vi "test_RemoteFgenSession_CallCloseMeasurementLinkSessionWithDetachBehavior_RemoteSessionDetached.vi"(8 "error in":errorcluster) -> (0 "error out":errorcluster, 2 "result":string, 3 "pass":bool)   [LabVIEW 2020, in "MeasurementServerTests.lvlib"]
uses:
  MeasurementServerTests.lvlib
  Runtime/Sessions/niFGEN Sessions/Session Factory/Session Factory.lvclass
  Runtime/Sessions/Instrument Sessions/ISession Factory/Initialize and Close Session Behavior.ctl
  Runtime/Sessions/Instrument Sessions/ISession Factory/ISession Factory.lvclass
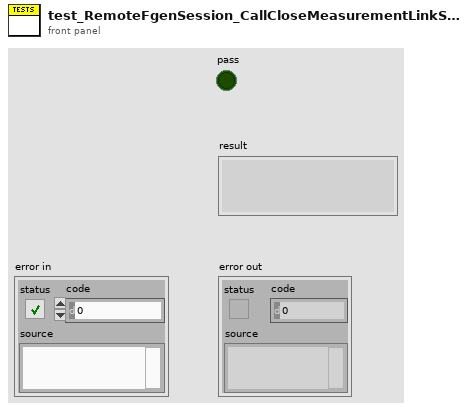
[diagram p1: front panel]
types:
  T1 = typedef "Plug-In SDK Instrument Sessions.lvlib/ISession Factory.lvclass/Remote Connection Options.ctl" = cluster{"session name":string, "address":string, "port":u32}
  T2 = typedef "Plug-In SDK Instrument Sessions.lvlib/ISession Factory.lvclass/Initialize and Close Session Behavior.ctl" = enum16{"Initialize and Close", "Attach and Detach", "Initialize and Detach", "Attach and Close"}
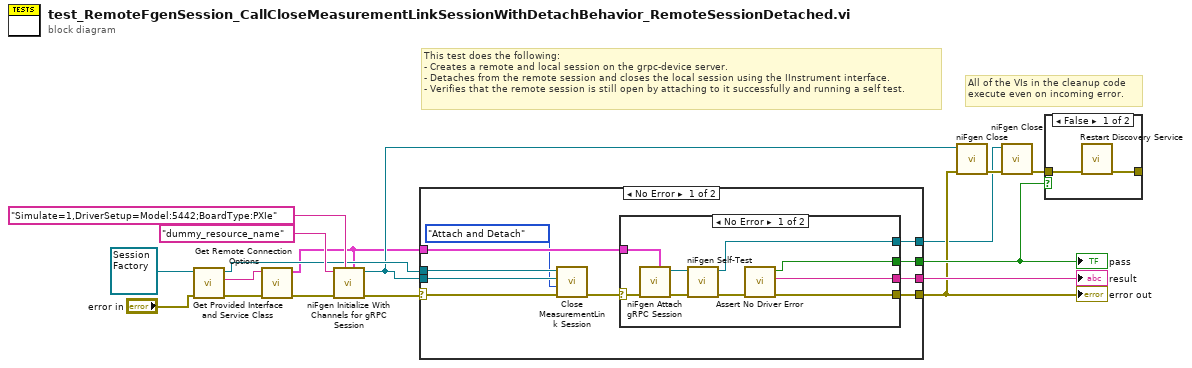
[diagram p0: block diagram]
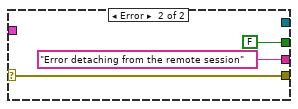
[diagram p2: hidden frame]
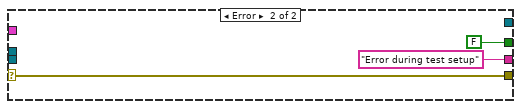
[diagram p3: hidden frame]
diagram:
  # "All of the VIs in the cleanup code\nexecute even on incoming error."
  # "This test does the following:\n- Creates a remote and local session on the grpc-device server.\n- Detaches from the remote session and closes the local session using the IInstrument interface.\n- Verifies that the remote session is still open by attaching to it successfully and running a self test."
  n1 = call-dynamic "Get Provided Interface and Service Class.vi"("error in"="error in", "session factory in"=refnum<class "Session Factory.lvclass"> refnum ("MeasurementLink niFGEN.lvlib:Instrument.lvclass")) -> ("error out"=w15:errorcluster, "provided interface"=w14:string, "session factory out"=w10:refnum<class "Session Factory.lvclass">)  [unwired: 6 in, 1 out]
  n2 = call "Get Remote Connection Options.vi"("error in"=w15, "provided interface"=w14) -> ("error out"=w16:errorcluster, "remote connection options"=w2:T1)  [unwired: 8 in]
  n3 = call <instrlib>:"niFgen Initialize With Channels for gRPC Session.vi"("gRPC Options"=w2, "Option String"="Simulate=1,DriverSetup=Model:5442;BoardType:PXIe" ("option string"), "error in (no error)"=w16, "Resource Name"="dummy_resource_name" ("resource name")) -> ("error out"=w11:errorcluster, "Instrument Handle Out"=w5:refnum<k15>)  [unwired: 6 in]
  n4 = case shown="No Error" w11 {
    selector: w11 -> [w27 w41]
    tunnel: w10 -> [w26 _]
    tunnel: w5 -> [w25 _]
    tunnel: w2 -> [w24 _]
    tunnel: [w22 w41] -> w4
    tunnel: [w21 FALSE] -> w6
    tunnel: [w20 "Error during test setup" ("f")] -> w9
    tunnel: [w18 _] -> w1
    frame No Error {
      n5 = call-dynamic "Close MeasurementLink Session.vi"("error in"=w27, "initialize and close session behavior"=Initialize_and_Close_Session_Behavior."Attach and Detach", "session in"=w25, "session factory in"=w26) -> ("error out"=w23:errorcluster)  [unwired: 7 in]
      n6 = case shown="No Error" w23 {
        selector: w23 -> [w36 w37]
        tunnel: w24 -> [w33 _]
        tunnel: [w28 w37] -> w22
        tunnel: [w30 FALSE] -> w21
        tunnel: [w29 "Error detaching from the remote session" ("f")] -> w20
        tunnel: [w32 _] -> w18
        frame No Error {
          n7 = call <instrlib>:"niFgen Attach gRPC Session.vi"("gRPC Options"=w33, "error in (no error)"=w36) -> ("error out"=w34:errorcluster, "Instrument Handle Out"=w35:refnum<k15>)  [unwired: 8 in]
          n8 = call <instrlib>:"niFgen Self-Test.vi"("error in (no error)"=w34, "Instrument Handle"=w35) -> ("error out"=w31:errorcluster, "Instrument Handle Out"=w32:refnum<k15>)  [unwired: 6 in, 2 out]
          n9 = call "Assert No Driver Error.vi"("error in"=w31) -> ("error out"=w28:errorcluster, "result"=w29:string, "pass?"=w30:bool)  [unwired: 8 in]
        }
        frame Error {
        }
      }
    }
    frame Error {
    }
  }
  "error out" <- w4
  "pass" <- w6
  "result" <- w9
  n10 = call <instrlib>:"niFgen Close.vi"("error in (no error)"=w4, "Instrument Handle"=w5) -> ("error out"=w8:errorcluster)  [unwired: 9 in]
  n11 = call <instrlib>:"niFgen Close.vi"("error in (no error)"=w8, "Instrument Handle"=w1) -> ("error out"=w7:errorcluster)  [unwired: 9 in]
  n12 = case shown="False" w6 {
    tunnel: [w44 _] -> _
    tunnel: w7 -> [w43 _]
    frame False {
      n13 = call "Restart Discovery Service.vi"("error in"=w43) -> ("error out"=w44:errorcluster)  [unwired: 10 in]
    }
    frame True {
    }
  }
